vi "Task.vi"(8 "error in (no error)":errorcluster, 11 "Group in":refnum<class "Group Config.lvclass">) -> (0 "error out":errorcluster, 2 "Task":refnum<class "Task Config.lvclass">, 3 "Group out":refnum<class "Group Config.lvclass">)   [LabVIEW 2020, in "VolatusConfig.lvlib" / "Group Config.lvclass"]
uses:
  Group Config.lvclass
  C:/dev/lv20CE/relink/lv-volatus/VolatusConfig/VolatusConfigElement/VolatusConfigElement.lvclass
  Task/Task Config.lvclass
  Meta Type.ctl
  VolatusConfigElement/VolatusConfigElement.lvclass/VolatusConfigElement.ctl
  VolatusConfigElement/Element.vi
  lv-cdm/CDM-Config/Config Lookup/Match Meta.vi
  lv-cdm/CDM-Config/Config Element/Owner.vi
  lv-cdm/CDM-Config/Config Filter/Config Lookup.lvclass
  Group Config.lvclass/Group Config.ctl
  VolatusConfigElement/VolatusConfigElement.lvclass
  VolatusConfig.lvlib
  C:/dev/lv20CE/relink/lv-volatus/VolatusConfig/Group/Group Config.lvclass
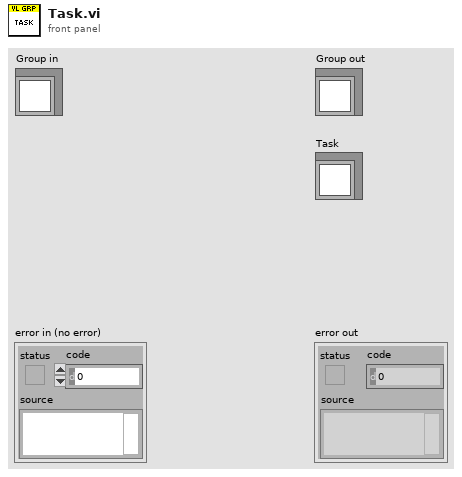
[diagram p1: front panel]
types:
  T1 = typedef "VolatusConfig.lvlib/Meta Type.ctl" = enum16{"UNKNOWN", "VL_System", "VL_Cluster", "VL_Node", "VL_Task", "VL_Group", "VL_Channel", "VL_Task_List", "VL_Scaling", "VL_Sensor", "VL_Sensor_List", "VL_Scale"}
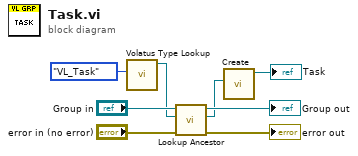
[diagram p0: block diagram]
diagram:
  n1 = call "Volatus Type Lookup.vi"("Meta Type"=Meta_Type."VL_Task") -> ("Config Lookup out"=w3:refnum<class "Config Lookup.lvclass">)  [unwired: 9 in, 1 out]
  n2 = call "Lookup Ancestor.vi"("error in (no error)"="error in (no error)", "Lookup"=w3, "VolatusConfigElement in"="Group in") -> ("error out"=→"error out":errorcluster, "Ancestor"=w2:refnum<class "Config Element.lvclass">, "VolatusConfigElement out"=→"Group out":refnum<class "Group Config.lvclass">)  [unwired: 6 in]
  n3 = call "Create.vi"("Element"=w2) -> ("Task out"=→"Task":refnum<class "Task Config.lvclass">)  [unwired: 9 in, 1 out]
